vi "Sort 2D String Array.vi"(0 "Calling VI Name":string, 1 "Column Sort Order":i32[](array[numeric]), 7 "Input Array":string[][](array[string]), 11 "Input Array Contains Header Row? (T)":T1=TRUE, 12 "Sort Ascending? (T)":T2=TRUE, 13 "Output Columns in Sort Order? (F)":bool, 14 "Preview Sorted Data? (F)":bool) -> (8 "Output Array":string[][](array[string]))   [LabVIEW 2010, in "xijk_select_best_filter.lvlib"]
doc: "Sort 2D String Array.vi\n\n<B>Description:</B>\n\nThis VI performs a multi-column sort on a 2D array of strings that contains both plain text strings and strings representing real numbers. The user can specify the column sort order.\n\nThis VI displays a busy indicator while the sort operation is in progress.\n\n<B>Usage:</B>\n\nWire all required inputs.\n\n<B>Inputs:</B>\n\nColumn Sort Order\n- This control specifies the column sort order. If it is left unwired, the sort order will be 0,1,2...\n\nCalling VI Name\n- This is the name of the VI that called the Sort 2D String Array VI.\n\nInput Array\n- This is the 2D array of strings containing plain text strings and strings representing real numbers that will be sorted.\n\nInput Array Contains Header Row? (T)\n- Set this input to True if the array to sort contains a header row.\n\nSort Ascending? (T)\n- Set this boolean False to perform a descending sort.\n\nOutput Columns in Sort Order? (F)\n- Set this boolean True to return the output data with the columns arranged in the order specified by the user. If set False, the columns in the output table are returned in their original positions.\n\nPreview Sorted Data? (F)\n- Set this input to True to enable the user to preview the sorted data.\n\n<B>Outputs:</B>\n\nOutput Array\n- This is the sorted 2D array of strings.\n\n<B>Developed by:</B>\n\nMark Ridgley\nmark.ridgley@logicpd.com"
uses:
  xijk_select_best_filter.lvlib
  _TypeDefs/TYPE - Sort Ascending.ctl
  _TypeDefs/TYPE - Input Array Contains Header Row.ctl
panel:
  out "Sorted Array":string[][](table)
  # "Number of columns in \"Input Array\" plus number of elements\nin \"Column Sort Order\" must be <= 256."
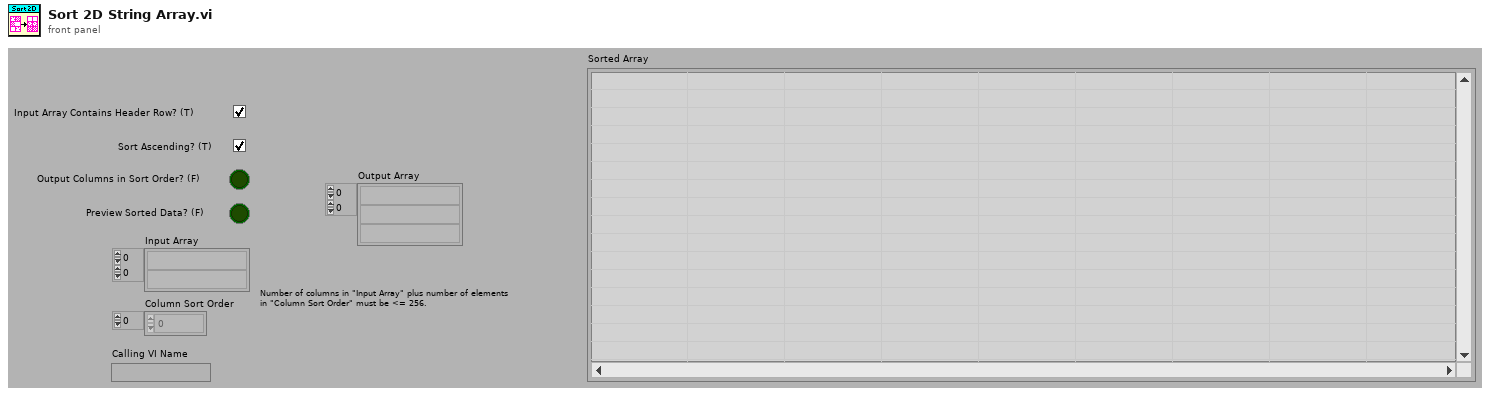
[diagram p1: front panel]
types:
  T1 = typedef "xijk_select_best_filter.lvlib/TYPE - Input Array Contains Header Row.ctl" = bool
  T2 = typedef "xijk_select_best_filter.lvlib/TYPE - Sort Ascending.ctl" = bool
  T3 = typedef "xijk_select_best_filter.lvlib/TYPE - Sorted Array (Cols in Original Order. Header row removed).ctl" = string[][]
  T4 = typedef "xijk_select_best_filter.lvlib/TYPE - Sorted Array (Cols in Sort Order. Header row removed).ctl" = string[][]
  T5 = typedef "xijk_select_best_filter.lvlib/TYPE - Sorted Array (Cols in Sort Order. Headers as last row).ctl" = string[][]
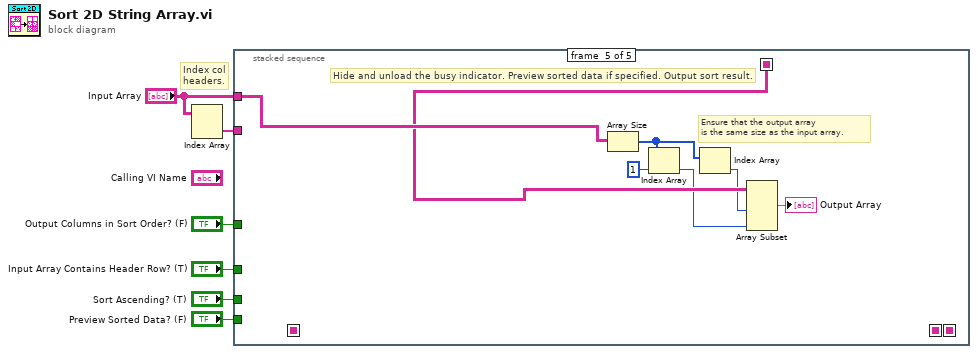
[diagram p0: block diagram]
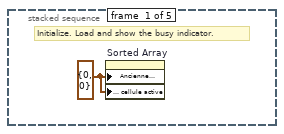
[diagram p2: hidden frame]
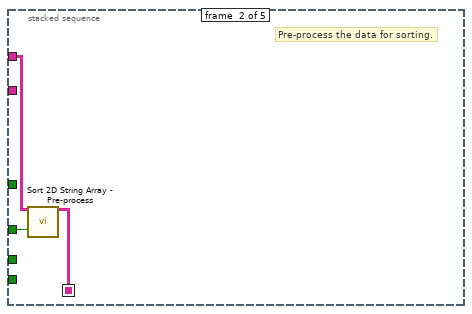
[diagram p3: hidden frame]
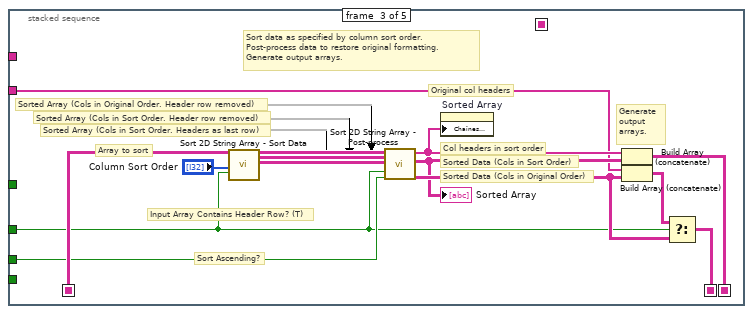
[diagram p4: hidden frame]
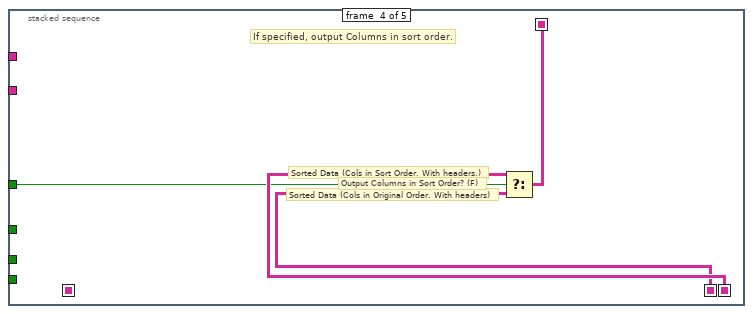
[diagram p5: hidden frame]
diagram:
  # "Index col\nheaders."
  n1 = Index Array(array="Input Array") -> (element=w4:string[])  [unwired: 2 in]
  n2 = stacked-sequence {
    seq-local: [_ w8 _ _ _] -> [_ _ w20 _ _]
    seq-local: [_ _ w14 _ _] -> [_ _ _ w27 _]
    seq-local: [_ _ w19 _ _] -> [_ _ _ w28 _]
    seq-local: [_ _ _ w25 _] -> [_ _ _ _ w34]
    tunnel: "Input Array" -> [_ w10 _ _ w35]
    tunnel: "Input Array Contains Header Row? (T)" -> [_ w9 w11 _ _]
    tunnel: w4 -> [_ _ w12 _ _]
    tunnel: "Sort Ascending? (T)" -> [_ _ w18 _ _]
    tunnel: "Output Columns in Sort Order? (F)" -> [_ _ _ w26 _]
    tunnel: "Preview Sorted Data? (F)" -> [_ _ _ _ _]
    frame #0 {
      w7 = cluster{i32, i32} {0, 0} ("Write Attribute")
      # "Initialize. Load and show the busy indicator."
      n3 = property on="Sorted Array" class="Tbl (strict)"("Ancienne position de modification"=w7, "Cellule active : cellule active"=w7) -> ()  [unwired: 2 in, 2 out]
    }
    frame #1 {
      # "Pre-process the data for sorting."
      n4 = call "Sort 2D String Array - Pre-process.vi"("Array to Sort In"=w10, "Input Array Contains Header Row? (T)"=w9) -> ("Array to Sort Out"=w8:string[][])  [unwired: 1 in, 16 out]
    }
    frame #2 {
      # "Sort Ascending?"
      # "Generate\noutput\narrays."
      # "Sort data as specified by column sort order.\nPost-process data to restore original formatting.\nGenerate output arrays."
      # "Original col headers"
      # "Input Array Contains Header Row? (T)"
      # "Sorted Array (Cols in Original Order. Header row removed)"
      # "Sorted Array (Cols in Sort Order. Header row removed)"
      # "Sorted Array (Cols in Sort Order. Headers as last row)"
      # "Sorted Data (Cols in Original Order)"
      # "Sorted Data (Cols in Sort Order)"
      # "Col headers in sort order"
      # "Array to sort"
      n5 = call "Sort 2D String Array - Sort Data.vi"("Array to sort in"=w20, "Column Sort Order"="Column Sort Order", "Input Array Contains Header Row? (T)"=w11) -> ("Sorted Array (Cols in Original Order. Header row removed)"=w21:T3, "Sorted Array (Cols in Sort Order. Header row removed)"=w24:T4, "Sorted Array (Cols in Sort Order. Headers as last row)"=w23:T5)  [unwired: 6 in, 8 out]
      n6 = call "Sort 2D String Array - Post-process.vi"("Sorted Array (Cols in Original Order. Header row removed)"=w21, "Sorted Array (Cols in Sort Order. Header row removed)"=w24, "Sorted Array (Cols in Sort Order. Headers as last row)"=w23, "Input Array Contains Header Row? (T)"=w11, "Sort Ascending? (T)"=w18) -> ("Column Headers (In Sort Order)"=w17:string[], "Sorted Data (Columns in Sort Order)"=w13:string[][], "Sorted Data (Columns in Original Order)"=w16:string[][])  [unwired: 5 in, 7 out]
      "Sorted Array" <- w13
      n7 = property on="Sorted Array" class="Tbl (strict)"("Chaînes d'en-tête de colonne []"=w17) -> ()  [unwired: 2 in, 2 out]
      n8 = Build Array (concatenate)(w17, w13) -> (w19:string[][])
      n9 = Build Array (concatenate)(w12, w16) -> (w15:string[][])
      n10 = Select(t=w15, s=w11, f=w16) -> (s? t:f=w14:string[][])
    }
    frame #3 {
      # "If specified, output Columns in sort order."
      # "Sorted Data (Cols in Original Order. With headers)"
      # "Sorted Data (Cols in Sort Order. With headers.)"
      # "Output Columns in Sort Order? (F)"
      n11 = Select(t=w28, s=w26, f=w27) -> (s? t:f=w25:string[][])
    }
    frame #4 {
      # "Ensure that the output array\nis the same size as the input array."
      # "Hide and unload the busy indicator. Preview sorted data if specified. Output sort result."
      n12 = Array Size(array=w35) -> (size(s)=w32:i32[])
      n13 = Index Array(array=w32, index=1) -> (element=w29:i32)
      n14 = Index Array(array=w32) -> (element=w30:i32)  [unwired: 1 in]
      n15 = Array Subset(array=w34, length (row)=w30, length (col)=w29) -> (→"Output Array":string[][])  [unwired: 2 in]
    }
  }
